vi "downconvert.vi"(5 "clock x2":refnum<k21>="Daughterboard 0\\Data Clock x2", 7 "reset":bool, 8 "input valid":bool, 10 "output sample rate":fxp<+,48,1>, 11 "data in":T1[](array[typedef])=[{"I"=0.0, "Q"=0.0, "overflow"=FALSE}, {"I"=0.0, "Q"=0.0, "overflow"=FALSE}]) -> (0 "output valid":bool, 3 "data out":T1[](array[typedef]))   [LabVIEW 2025]
uses:
  <instrlib>/_niInstr/DSP/v1/Shared/Public/IQ Data.ctl
  <instrlib>/_niInstr/DSP/v1/FPGA/Public/Sub VIs/Fractional Decimator/Fractional Decimator - 1 spc - 2x oc.vi
  <instrlib>/_niInstr/DSP/v1/XNodes/Public/Decimator/niInstr DSP v1 Decimator FPGA.xnode
  <instrlib>/_niInstr/DSP/v1/Shared/niInstr DSP v1 Shared.lvlib
  <instrlib>/_niInstr/DSP/v1/FPGA/niInstr DSP v1 FPGA.lvlib
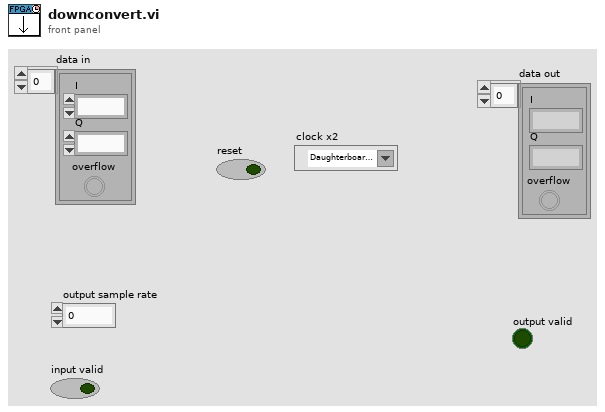
[diagram p1: front panel]
types:
  T1 = typedef "niInstr DSP v1 Shared.lvlib/IQ Data.ctl" = cluster{"I":fxp<+/-,18,1>, "Q":fxp<+/-,18,1>, "overflow":bool}
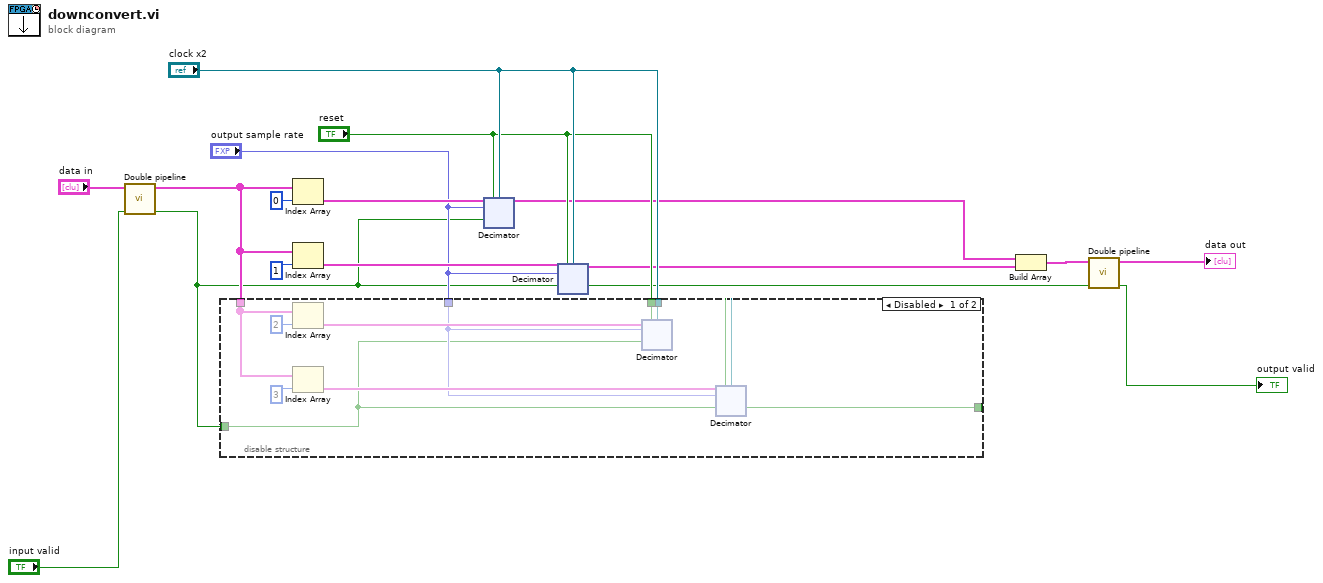
[diagram p0: block diagram]
diagram:
  n1 = call "Double pipeline.vi"("input valid"="input valid", "data in"="data in") -> ("input valid pipe"=w2:bool, "data in pipe"=w4:T1[])  [unwired: 8 in]
  n2 = disable-structure shown="Disabled" {
    disable-tunnel: "clock x2" -> [w25 _]
    disable-tunnel: "reset" -> [w24 w48]
    disable-tunnel: "output sample rate" -> [w23 _]
    disable-tunnel: [w20 w48] -> _
    disable-tunnel: w4 -> [w19 _]
    disable-tunnel: w2 -> [w18 _]
    frame Disabled {
      n3 = Index Array(array=w19, index=2) -> (element=w26:T1)
      n4 = Index Array(array=w19, index=3) -> (element=w27:T1)
      n5 = xnode "Decimator"("data in"=w26, "reset"=w24, "input valid"=w18, "output sample rate"=w23, "clock x2"=w25) -> ("data out"=w21:T1)  [unwired: 1 in, 2 out]
      n6 = xnode "Decimator"("data in"=w27, "reset"=w24, "input valid"=w18, "output sample rate"=w23, "clock x2"=w25) -> ("data out"=w22:T1, "output valid"=w20:bool)  [unwired: 1 in, 1 out]
    }
    frame Enabled {
    }
  }
  n7 = Index Array(array=w4, index=0) -> (element=w15:T1)
  n8 = Index Array(array=w4, index=1) -> (element=w14:T1)
  n9 = xnode "Decimator"("data in"=w15, "reset"="reset", "input valid"=w2, "output sample rate"="output sample rate", "clock x2"="clock x2") -> ("data out"=w10:T1)  [unwired: 1 in, 2 out]
  n10 = xnode "Decimator"("data in"=w14, "reset"="reset", "input valid"=w2, "output sample rate"="output sample rate", "clock x2"="clock x2") -> ("data out"=w9:T1, "output valid"=w1:bool)  [unwired: 1 in, 1 out]
  n11 = Build Array(w10, w9) -> (w8:T1[])
  n12 = call "Double pipeline.vi"("input valid"=w1, "data in"=w8) -> ("input valid pipe"=→"output valid":bool, "data in pipe"=→"data out":T1[])  [unwired: 8 in]
